vi "Analyze Image.vi"(8 "error in (no error)":errorcluster, 9 "Image Nr.":i32, 10 "Pre Procesed Image":T1, 11 "HIJ Vision Camera App in":refnum<class "HIJ Vision Camera App.lvclass">) -> (0 "error out":errorcluster, 3 "HIJ Vision Camera App out":refnum<class "HIJ Vision Camera App.lvclass">)   [LabVIEW 2020, in "HIJ Vision Camera App.lvlib" / "HIJ Vision Camera App.lvclass"]
uses:
  HIJ Vision Camera App.lvclass
  HIJ Vision Application/HIJ Vision Application/HIJ Vision Application.lvclass
  <vilib>/vision/Image Controls.llb/IMAQ Image.ctl
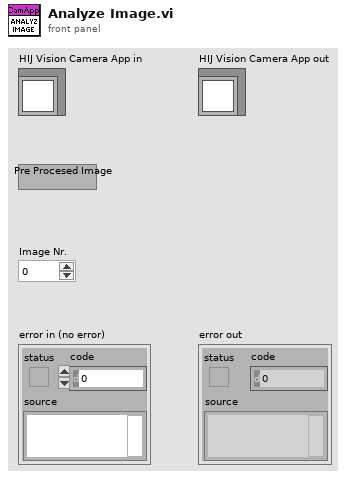
[diagram p1: front panel]
types:
  T1 = typedef "IMAQ Image.ctl" = refnum<image>
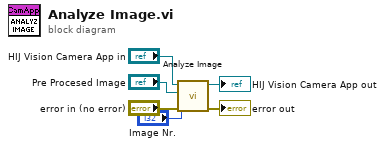
[diagram p0: block diagram]
diagram:
  n1 = call-parent "Analyze Image.vi"("error in (no error)"="error in (no error)", "Image Nr."="Image Nr.", "Pre Procesed Image"="Pre Procesed Image", "HIJ Vision Application in"="HIJ Vision Camera App in") -> ("error out"=→"error out":errorcluster, "HIJ Vision Application out"=→"HIJ Vision Camera App out":refnum<class "HIJ Vision Camera App.lvclass">)  [unwired: 6 in]
